vi "Bundle.vi"(7 "Instrument ID":u32, 8 "Pre Initialization Data":variant, 9 "Connection Type":T1=enum."SwitchBlock Device", 10 "Alias":string, 11 "Driver Path":path) -> (3 "Register Instrument Msg out":refnum<class "Register Instrument Msg.lvclass">)   [LabVIEW 2020, in "Instrument Handler.lvlib" / "Register Instrument Msg.lvclass"]
doc: "Populate the Register Instrument Msg."
uses:
  Register Instrument Msg.lvclass
  PPL/HDH.Actor Framework.Core.Instrument Driver.lvlibp/Instrument Driver/Controls/Ctl_ConnectionType.ctl
  Register Instrument Msg.lvclass/Register Instrument Msg.ctl
  PPL/HDH.Actor Framework.Core.Instrument Driver.lvlibp/Instrument Driver/Instrument Driver.lvclass
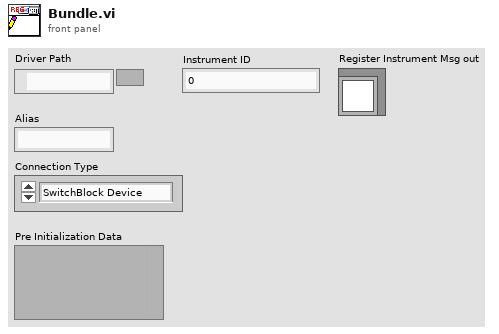
[diagram p1: front panel]
types:
  T1 = typedef "HDH.Actor Framework.Core.Instrument Driver.lvlibp/Instrument Driver.lvclass/Ctl_ConnectionType.ctl" = enum16{"BuiltIn/System", "PXI/PCI", "USB", "GPIB", "VXI", "Serial", "TCP/IP", "cRIO", "SCXI", "cDAQ", "SwitchBlock", "SCC", "FireWire", "Accessory", "CAN", "SwitchBlock Device"}
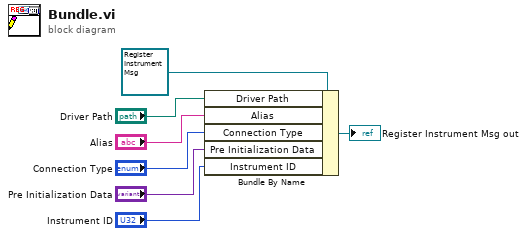
[diagram p0: block diagram]
diagram:
  n1 = Bundle By Name(cluster=refnum<class "Register Instrument Msg.lvclass"> refnum ("Register Instrument Msg in"), "Driver Path"="Driver Path", "Alias"="Alias", "Connection Type"="Connection Type", "Pre Initialization Data"="Pre Initialization Data", "Instrument ID"="Instrument ID") -> (→"Register Instrument Msg out":refnum<class "Register Instrument Msg.lvclass">)
